vi "about.vi"(8 "error in (no error)":errorcluster) -> (0 "error out":errorcluster)   [LabVIEW 2015, in "ESLSCDLL.lvlib"]
uses:
  ESLSCDLL.lvlib
  Globals.vi
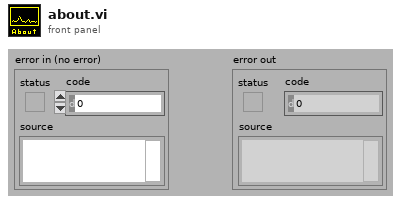
[diagram p1: front panel]
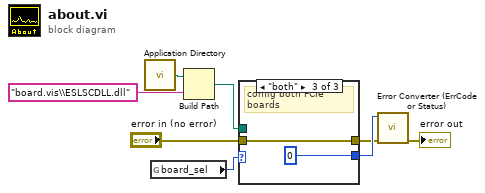
[diagram p0: block diagram]
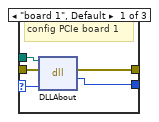
[diagram p2: hidden frame]
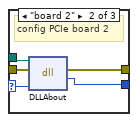
[diagram p3: hidden frame]
diagram:
  n1 = call <vilib>:"Application Directory.vi"() -> ("Application Directory"=w3:path)
  n2 = global read "Globals.vi" "board_sel"() -> (w4:enum32{"0", "board 1", "board 2", "both"})
  n3 = Build Path(base path=w3, name or relative path="board.vis\\ESLSCDLL.dll") -> (appended path=w1:path)
  n4 = case shown="\"both\"" w4 {
    selector: w4 -> [w13 w18 _]
    tunnel: [w12 w17 0 ("es_status_codes")] -> w8
    tunnel: "error in (no error)" -> [w11 w16 w19]
    tunnel: [w10 w15 w19] -> w5
    tunnel: w1 -> [w9 w14 _]
    frame "board 1", Default {
      # "config PCIe board 1"
      n5 = dll-call lib="C:/ENTW/PCIE/LV64/board.vis/ESLSCDLL.dll" fn="DLLAbout" ("lwlscdll.dll:DLLAboutDrv")(path in=w9, error in=w11, "drv"=w13) -> (error out=w10:errorcluster, "es_status_codes"=w12:i32)  [unwired: 2 in, 1 out]
    }
    frame "board 2" {
      # "config PCIe board 2"
      n6 = dll-call lib="C:/ENTW/PCIE/LV64/board.vis/ESLSCDLL.dll" fn="DLLAbout" ("lwlscdll.dll:DLLAboutDrv")(path in=w14, error in=w16, "drv"=w18) -> (error out=w15:errorcluster, "es_status_codes"=w17:i32)  [unwired: 2 in, 1 out]
    }
    frame "both" {
      # "config both PCIe boards"
    }
  }
  n7 = call "Error Converter (ErrCode or Status).vi"("error in (no error)"=w5, "error code"=w8) -> ("error out"=→"error out":errorcluster)  [unwired: 9 in]
